vi "To JSON.vi"(6 "Pretty Print?":bool, 8 "error in (no error)":errorcluster, 11 "Type in":refnum<class "Abs_Waveform.lvclass">) -> (0 "error out":errorcluster, 2 "JSON":string, 3 "Type out":refnum<class "Abs_Waveform.lvclass">)   [LabVIEW 2021, in "Abs_Waveform.lvclass"]
uses:
  Abs_Waveform.lvclass
  C:/Program Files (x86)/National Instruments/LabVIEW 2021/vi.lib/TSA/Abstract Data Classes/Abs_Types/Type/Abs_Type.lvclass
  e8ef0cb7-7174-41be-ae40-fa79b1513943.vi
  <vilib>/Utility/LVClass/Get LV Class Name.vi
  <vilib>/JDP Science/JSONtext/Variant to JSON Text.vi
  <vilib>/JDP Science/JSONtext/Set Multiple Object Items.vi
  Value/Abs_Value.lvclass
  <vilib>/JDP Science/JSONtext/LVClass Serializer/JSONtext LVClass Serializer.lvclass
  Type/Abs_Type.lvclass
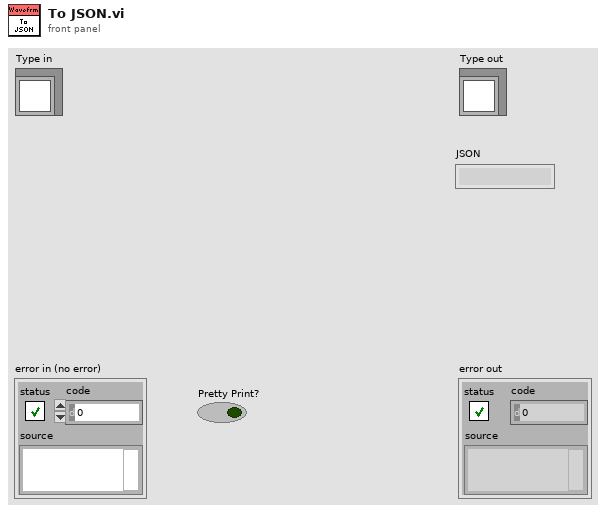
[diagram p1: front panel]
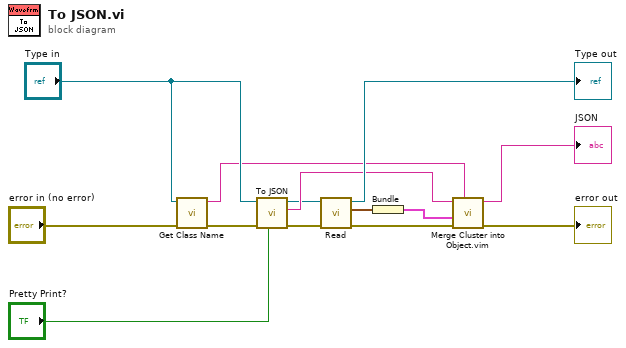
[diagram p0: block diagram]
diagram:
  n1 = call "Get Class Name.vi"("error in (no error)"="error in (no error)", "Abs_Type in"="Type in") -> ("error out"=w4:errorcluster, "class name"=w6:string)  [unwired: 8 in]
  n2 = call-parent "To JSON.vi"("Pretty Print?"="Pretty Print?", "error in (no error)"=w4, "Type in"="Type in") -> ("error out"=w3:errorcluster, "JSON"=w5:string, "Type out"=w1:refnum<class "Abs_Waveform.lvclass">)  [unwired: 6 in]
  n3 = call-dynamic "Read.vi"("error in (no error)"=w3, "Abs_Waveform in"=w1) -> ("error out"=w2:errorcluster, "Waveform"=w7:waveform(dbl), "Abs_Waveform out"=→"Type out":refnum<class "Abs_Waveform.lvclass">)  [unwired: 7 in]
  n4 = Bundle("Waveform"=w7) -> (w8:cluster{"Waveform":waveform(dbl)})  [unwired: 1 in]
  n5 = call "Merge Cluster into Object.vim"("$Path or Item Name"=w6, "error in (no error)"=w2, "Any Cluster"=w8, "JSON"=w5) -> ("error out"=→"error out":errorcluster, "<JSON>"=→"JSON":string)  [unwired: 5 in]
